vi "Write to Hardware.vi"(8 "error in":errorcluster, 9 "trigger values":dbl[](array[numeric]), 10 "Values in":dbl[](array[numeric]), 11 "Ballard ARINC-429 Tx Execution Unit in":refnum<class "Tx Scheduled Labels Execution Unit.lvclass">) -> (0 "error out":errorcluster, 1 "trigger values out":dbl[](array[numeric]), 2 "Values out":dbl[](array[numeric]), 3 "Ballard ARINC-429 Tx Execution Unit out":refnum<class "Tx Scheduled Labels Execution Unit.lvclass">)   [LabVIEW 2020, in "Ballard ARINC 429 Engine.lvlib" / "Implementation.lvlib" / "Tx Scheduled Labels Execution Unit.lvclass"]
uses:
  Tx Scheduled Labels Execution Unit.lvclass
  Execution Unit/Execution Unit.lvclass
  <instrlib>/BTI429Lib/BTI429LV.lvlib
  Custom Device/Custom Device.lvlib
  C:/Users/Administrator/Desktop/GIT/niveristand-ballard-arinc429-custom-device/Source/Custom Device Support/Engine/Implementation/Execution Unit/Execution Unit.lvclass
  C:/Users/Administrator/Desktop/GIT/niveristand-ballard-arinc429-custom-device/Source/Custom Device Support/Engine/Interfaces/Execution Unit/Execution Unit.lvclass
  C:/Users/Administrator/Desktop/GIT/niveristand-ballard-arinc429-custom-device/Source/Custom Device Support/Engine/Implementation/Tx Scheduled Labels Execution Unit/Tx Scheduled Labels Execution Unit.lvclass
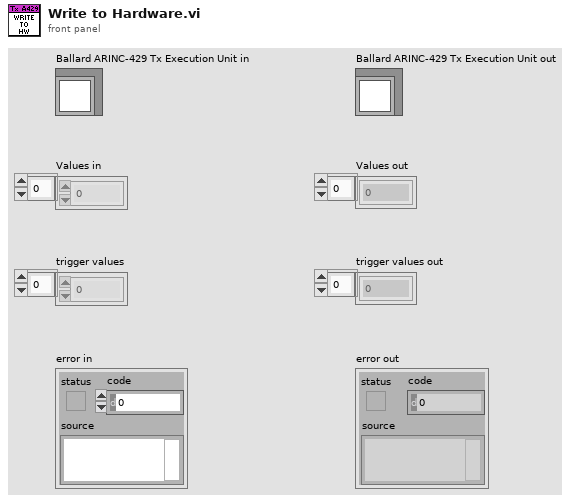
[diagram p1: front panel]
types:
  T1 = typedef "Map of Values Indexes to Channel and Label Indexes.ctl" = map{i32, cluster{"channel index":i32, "label index":i32, "group values start index":i32, "values in group":i32}}
  T2 = typedef "RT Hardware Channel Settings.ctl" = cluster{"channel #":u16, "channel handle":u64, "labels settings for RT":T3[]}
  T3 = typedef "RT Label Settings.ctl" = cluster{"Name":string, "xmlName":string, "label":T4, "transfer period":u32, "SDI_Enabled":bool, "SDI":u8, "parameter driver data":T5, "transfer type":T9, "has timestamp?":bool, "Label Disable/Trigger Channel Reference":T8, "Message Handle":u64, "Initialized?":bool, "Word Initial Raw Value":u32, "Label Timestamp Channel Data Reference":T10, "disabled":bool}
  T4 = typedef "Label.ctl" = u8
  T5 = typedef "RT Parameters.ctl" = cluster{"parameter definitions":T6[], "Tx parameter refs":T8[]}
  T6 = typedef "Parameter Definition.ctl" = cluster{"start index":i32, "size":i32, "encoding":T7, "signed":bool, "scale multiplier":dbl, "scale offset":dbl}
  T7 = typedef "Encoding and Decoding.lvlib/Encoding.ctl" = enum16{"BNR", "BCD", "Discrete"}
  T8 = typedef "Custom Device API.lvlib/Custom Device Item Ref.ctl" = u64
  T9 = typedef "Transfer Type.ctl" = enum16{"Scheduled", "Acyclic", "Block", "Strobe"}
  T10 = typedef "Custom Device API.lvlib/Data Reference.ctl" = i32
  T11 = cluster{"channel index":i32, "label index":i32, "group values start index":i32, "values in group":i32}
  T12 = typedef "Ballard ARINC 429 Engine.lvlib/Custom Device.lvlib/Hardware Handles.ctl" = cluster{"core handle":u64, "core reader handle":u64, "channel handles":u64[]}
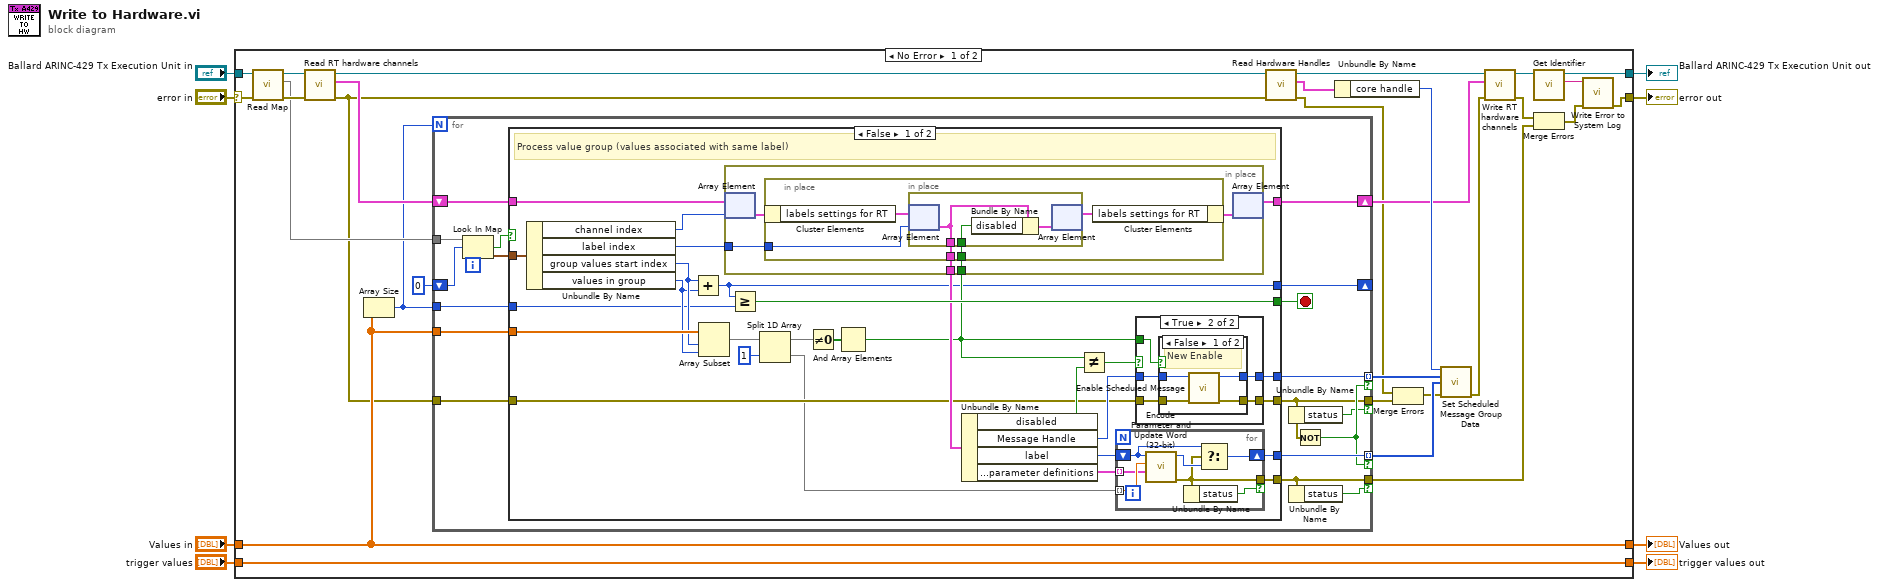
[diagram p0: block diagram]
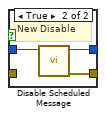
[diagram p3: hidden frame]
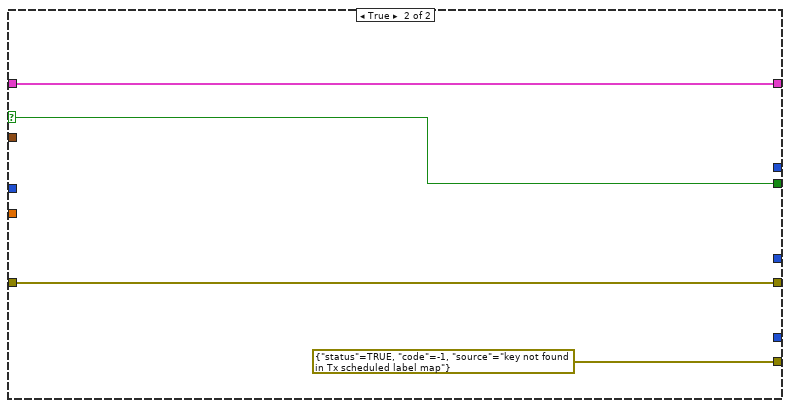
[diagram p4: hidden frame]
diagram:
  n1 = case shown="No Error" "error in" {
    selector: "error in" -> [w30 w123]
    tunnel: [w10 w123] -> w8
    tunnel: [w26 w122] -> w6
    tunnel: "Values in" -> [w26 w122]
    tunnel: [w12 w124] -> w4
    tunnel: "Ballard ARINC-429 Tx Execution Unit in" -> [w31 w124]
    tunnel: [w15 w121] -> w2
    tunnel: "trigger values" -> [w15 w121]
    frame No Error {
      n2 = call "Read Map.vi"("error in"=w30, "Ballard ARINC-429 Tx Execution Unit in"=w31) -> ("error out"=w29:errorcluster, "map from values indexes to RT info indexes"=w28:T1, "Ballard ARINC-429 Tx Execution Unit out"=w32:refnum<class "Tx Scheduled Labels Execution Unit.lvclass">)  [unwired: 7 in]
      n3 = call "Read RT hardware channels.vi"("error in"=w29, "Ballard ARINC-429 Tx Execution Unit in"=w32) -> ("error out"=w21:errorcluster, "RT hardware channels"=w34:T2[], "Ballard ARINC-429 Tx Execution Unit out"=w37:refnum<class "Tx Scheduled Labels Execution Unit.lvclass">)  [unwired: 7 in]
      n4 = Array Size(array=w26) -> (size(s)=w25:i32)
      n5 = for {
        N: w25 -> [_]
        tunnel: w26 -> [w49]
        tunnel: [w55] -> w17 mode=indexing if=w42
        tunnel: [w54] -> w33 mode=indexing if=w42
        tunnel: w28 -> [w52]
        shift-right: [w47] -> _
        shift-left: 0 -> [w51]
        tunnel: w25 -> [w48]
        shift-right: [w44] -> w24
        shift-left: w34 -> [w53]
        tunnel: w21 -> [w43]
        tunnel: [w39] -> w20 if=w38
        tunnel: [w41] -> w18 if=w40
        stop <- w45 stop-if-true
        n6 = Look In Map(map=w52, key=w51) -> (key not found?=w46:bool, value=w50:T11)  [unwired: 1 in]
        n7 = case shown="False" w46 {
          selector: w46 -> [_ w120]
          tunnel: [w77 _] -> w55
          tunnel: w43 -> [w58 w118]
          tunnel: [w56 errorcluster {"status"=TRUE, "code"=-1, "source"="key not found in Tx scheduled label map"} ("error in")] -> w41
          tunnel: [w67 _] -> w54
          tunnel: w53 -> [w62 w119]
          tunnel: w50 -> [w83 _]
          tunnel: w49 -> [w82 _]
          tunnel: w48 -> [w79 _]
          tunnel: [w63 _] -> w47
          tunnel: [w78 w120] -> w45
          tunnel: [w60 w119] -> w44
          tunnel: [w59 w118] -> w39
          frame False {
            # "Process value group (values associated with same label)"
            n8 = Unbundle By Name(w83) -> ("channel index"=w61:i32, "label index"=w64:i32, "group values start index"=w81:i32, "values in group"=w80:i32)
            n9 = Add(x=w81, y=w80) -> (x+y=w63:i32)
            n10 = Array Subset(array=w82, index=w81, length=w80) -> (w75:dbl[])
            n11 = Greater Or Equal?(x=w63, y=w79) -> (x >= y?=w78:bool)
            n12 = Split 1D Array(array=w75, index=1) -> (first subarray=w74:dbl[], second subarray=w57:dbl[])
            n13 = Not Equal To 0?(x=w74) -> (x != 0?=w73:bool[])
            n14 = And Array Elements(Boolean array=w73) -> (logical AND=w65:bool)
            n15 = in-place {
              in-place-border: [w88] -> w66
              in-place-border: w65 -> [w87]
              in-place-border: w64 -> [w86]
              n16 = in-place-array #1(w62, w61) -> (w84:T2)
              n17 = in-place {
                in-place-border: [w93] -> w88
                in-place-border: w87 -> [w92]
                in-place-border: w86 -> [w91]
                n18 = in-place-cluster #2(w84) -> ("labels settings for RT"=w90:T3[])
                n19 = in-place {
                  in-place-border: [w95] -> w93
                  in-place-border: w92 -> [w96]
                  n20 = in-place-array #3(w90, w91) -> (w95:T3)
                  n21 = Bundle By Name(cluster=w95, "disabled"=w96) -> (w94:T3)
                  n22 = in-place-array #3(w94) -> (w89:T3[])  [unwired: 1 out]
                }
                n23 = in-place-cluster #2("labels settings for RT"=w89) -> (w85:T2)
              }
              n24 = in-place-array #1(w85) -> (w60:T2[])  [unwired: 1 out]
            }
            n25 = Unbundle By Name(w66) -> ("disabled"=w69:bool, "Message Handle"=w68:u64, "label"=w71:T4, "parameter driver data.parameter definitions"=w72:T6[])
            n26 = Not Equal?(x=w65, y=w69) -> (x != y?=w70:bool)
            n27 = for {
              tunnel: w57 -> [w116] mode=indexing
              shift-right: [w113] -> w77
              shift-left: w71 -> [w114]
              tunnel: w72 -> [w115] mode=indexing
              tunnel: [w111] -> w56 if=w110
              n28 = call "Encode Parameter and Update Word (32-bit).vi"("parameter definition"=w115, "parameter value"=w116, "word in"=w114) -> ("error out"=w111:errorcluster, "word out"=w112:u32)  [unwired: 7 in]
              n29 = Unbundle By Name(w111) -> ("status"=w110:bool)
              n30 = Select(t=w114, s=w111, f=w112) -> (s? t:f=w113:u32)
            }
            n31 = case shown="True" w70 {
              tunnel: w65 -> [_ w102]
              tunnel: w68 -> [w97 w101]
              tunnel: [w97 w100] -> w67
              tunnel: [_ w99] -> w59
              tunnel: w58 -> [_ w98]
              frame False {
              }
              frame True {
                n32 = case shown="False" w102 {
                  tunnel: w101 -> [w106 w109]
                  tunnel: [w105 w107] -> w99
                  tunnel: [w104 w108] -> w100
                  tunnel: w98 -> [w103 _]
                  frame False {
                    # "New Enable"
                    n33 = call <instrlib>:"Enable Scheduled Message.vi"("error in (no error)"=w103, "message handle in"=w106) -> ("error out"=w105:errorcluster, "message handle out"=w104:u64)  [unwired: 8 in]
                  }
                  frame True {
                    # "New Disable"
                    n34 = call <instrlib>:"Disable Scheduled Message.vi"("message handle in"=w109) -> ("error out"=w107:errorcluster, "message handle out"=w108:u64)  [unwired: 9 in]
                  }
                }
              }
            }
          }
          frame True {
          }
        }
        n35 = Unbundle By Name(w39) -> ("status"=w38:bool)
        n36 = Unbundle By Name(w41) -> ("status"=w40:bool)
        n37 = Not(x=w39) -> (.not. x?=w42:bool)
      }
      n38 = call "Read Hardware Handles.vi"("error in"=w21, "Ballard ARINC-429 Execution Unit in"=w37) -> ("error out"=w19:errorcluster, "hardware handles"=w36:T12, "Ballard ARINC-429 Execution Unit out"=w23:refnum<class "Tx Scheduled Labels Execution Unit.lvclass">)  [unwired: 7 in]
      n39 = Unbundle By Name(w36) -> ("core handle"=w35:u64)
      n40 = Merge Errors(w19, w20) -> (w16:errorcluster)
      n41 = call <instrlib>:"Set Scheduled Message Group Data.vi"("core handle in"=w35, "message handles in"=w33, "values"=w17, "error in (no error)"=w16) -> ("error out"=w22:errorcluster)  [unwired: 8 in, 3 out]
      n42 = call "Write RT hardware channels.vi"("error in"=w22, "RT hardware channels"=w24, "Ballard ARINC-429 Tx Execution Unit in"=w23) -> ("error out"=w9:errorcluster, "Ballard ARINC-429 Tx Execution Unit out"=w13:refnum<class "Tx Scheduled Labels Execution Unit.lvclass">)  [unwired: 7 in]
      n43 = call-dynamic "Get Identifier.vi"("Ballard ARINC-429 Execution Unit in"=w13) -> ("identifier"=w14:string, "Ballard ARINC-429 Execution Unit out"=w12:refnum<class "Tx Scheduled Labels Execution Unit.lvclass">)  [unwired: 8 in, 1 out]
      n44 = Merge Errors(w9, w18) -> (w11:errorcluster)
      n45 = call "Write Error to System Log.vi"("error in"=w11, "identifier"=w14) -> ("error out"=w10:errorcluster)  [unwired: 9 in]
    }
    frame Error {
    }
  }
  "error out" <- w8
  "Ballard ARINC-429 Tx Execution Unit out" <- w4
  "Values out" <- w6
  "trigger values out" <- w2
